vi "Get Message.vi"(8 "error in (no error)":errorcluster, 11 "SPARC4_GUI in":refnum<class "SPARC4_GEI.lvclass">) -> (0 "error out":errorcluster, 3 "SPARC4_GUI out":refnum<class "SPARC4_GEI.lvclass">)   [LabVIEW 2018, in "SPARC4_GEI.lvclass"]
uses:
  SPARC4_GEI.lvclass
  SPARC4_GEI.lvclass/SPARC4_GEI.ctl
  Channel GUI/Channel GEI.lvclass
  RxTx/RxTx.lvclass
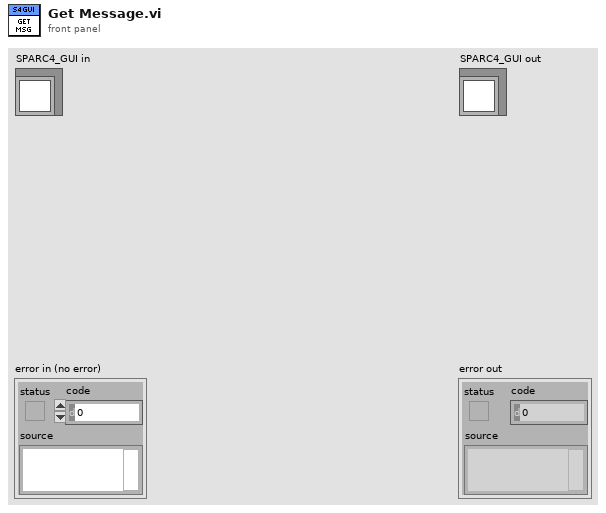
[diagram p1: front panel]
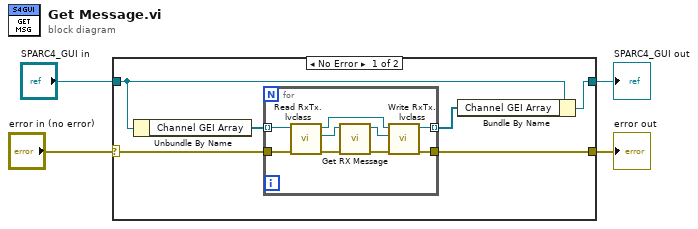
[diagram p0: block diagram]
diagram:
  n1 = case shown="No Error" "error in (no error)" {
    selector: "error in (no error)" -> [w6 w21]
    tunnel: [w8 w21] -> w3
    tunnel: [w9 w20] -> w1
    tunnel: "SPARC4_GUI in" -> [w10 w20]
    frame No Error {
      n2 = Unbundle By Name(w10) -> ("Channel GEI Array"=w7:refnum<class "Channel GEI.lvclass">[])
      n3 = for {
        tunnel: [w13] -> w8
        tunnel: w7 -> [w16] mode=indexing
        tunnel: w6 -> [w15]
        tunnel: [w14] -> w5 mode=indexing
        n4 = call "Read RxTx.lvclass.vi"("error in (no error)"=w15, "Channel GUI in"=w16) -> ("error out"=w19:errorcluster, "RxTx.lvclass"=w18:refnum<class "RxTx.lvclass">, "Channel GUI out"=w17:refnum<class "Channel GEI.lvclass">)  [unwired: 7 in]
        n5 = call "Get RX Message.vi"("error in (no error)"=w19, "RxTx in"=w18) -> ("error out"=w12:errorcluster, "RxTx out"=w11:refnum<class "RxTx.lvclass">)  [unwired: 8 in]
        n6 = call "Write RxTx.lvclass.vi"("error in (no error)"=w12, "RxTx.lvclass"=w11, "Channel GUI in"=w17) -> ("error out"=w13:errorcluster, "Channel GUI out"=w14:refnum<class "Channel GEI.lvclass">)  [unwired: 7 in]
      }
      n7 = Bundle By Name(cluster=w10, "Channel GEI Array"=w5) -> (w9:refnum<class "SPARC4_GEI.lvclass">)
    }
    frame Error {
    }
  }
  "error out" <- w3
  "SPARC4_GUI out" <- w1
